vi "Main.vi"(11 "Args":string[](array[string])) -> (2 "Output":string, 3 "Exit Code":i32)   [LabVIEW 2021]
uses:
  <vilib>/Utility/config.llb/Read Key (String).vi
  <vilib>/Utility/file.llb/Write Delimited Spreadsheet (string).vi
  <vilib>/Utility/config.llb/Read Key (U32).vi
  Add_Library.lvlib
  <vilib>/Utility/config.llb/NI_LVConfig.lvlib
panel:
  in  "y":u64[](array[numeric])=[1, 2, 3]
  in  "x":u64[](array[numeric])=[1, 2, 3]
  out "x+y":u64[](array[numeric])
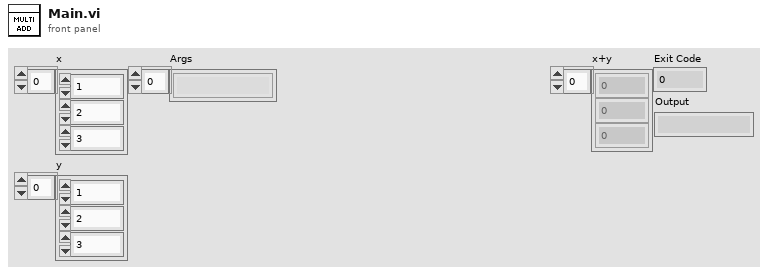
[diagram p1: front panel]
types:
  T1 = typedef "NI_LVConfig.lvlib/Config Data RefNum.ctl" = refnum<k1>
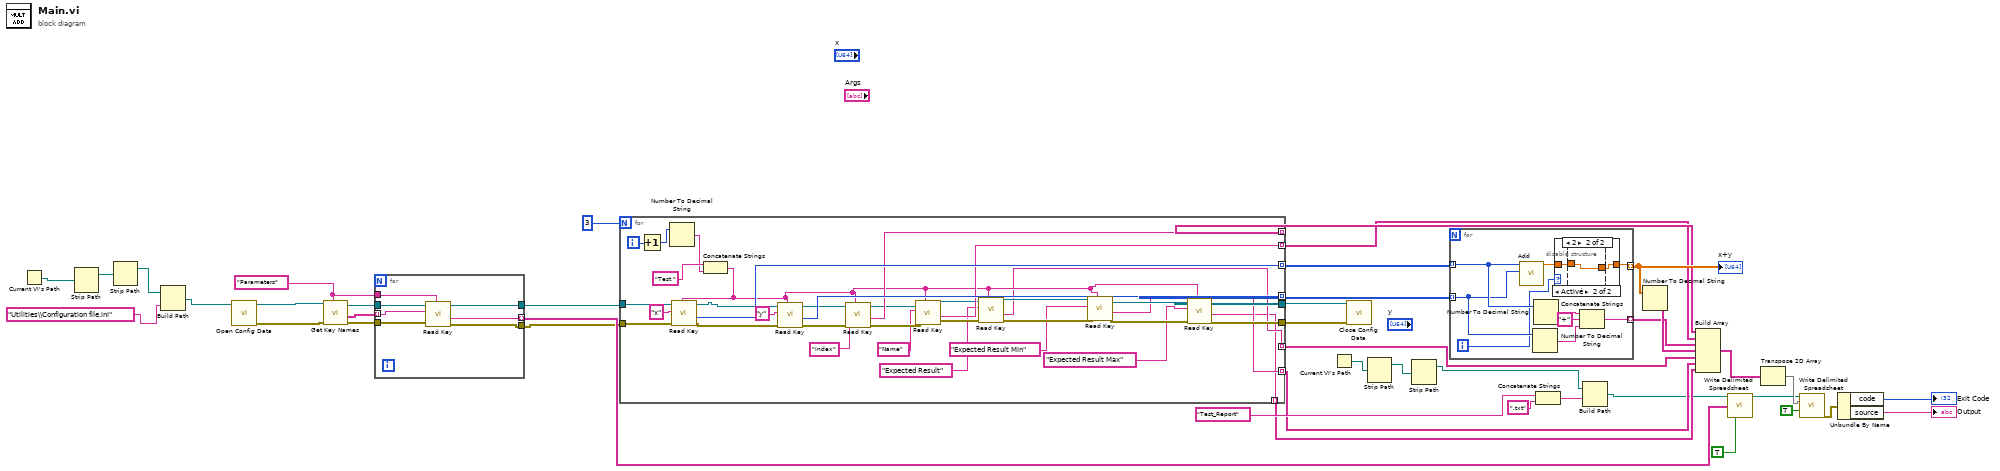
[diagram p0: block diagram]
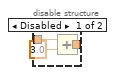
[diagram p3: hidden frame]
diagram:
  w8 = "Parameters" ("section")
  n1 = Current VI's Path() -> (path=w29:path)
  n2 = Strip Path(path=w29) -> (stripped path=w28:path)  [unwired: 1 out]
  n3 = Strip Path(path=w28) -> (stripped path=w27:path)  [unwired: 1 out]
  n4 = Build Path(base path=w27, name or relative path="Utilities\\Configuration file.ini" ("Report Path")) -> (appended path=w25:path)
  n5 = call <vilib>:"Open Config Data.vi"("configuration file path"=w25) -> ("error out"=w13:errorcluster, "refnum"=w14:T1)  [unwired: 8 in, 1 out]
  n6 = call <vilib>:"Get Key Names.vi"("section"=w8, "error in (no error)"=w13, "refnum"=w14) -> ("error out"=w10:errorcluster, "key names"=w9:string[], "refnum out"=w12:T1)  [unwired: 5 in, 1 out]
  n7 = for {
    tunnel: w12 -> [w49]
    tunnel: [w48] -> w11
    tunnel: w10 -> [w47]
    tunnel: w9 -> [w46] mode=indexing
    tunnel: w8 -> [w45]
    tunnel: [w44] -> w3 mode=indexing
    tunnel: [w43] -> w2
    n8 = call-poly <vilib>:"Read Key.vi"("section"=w45, "error in (no error)"=w47, "key"=w46, "refnum"=w49) -> ("error out"=w43:errorcluster, "value"=w44:string, "refnum out"=w48:T1)  [unwired: 4 in, 1 out]
  }
  n9 = for {
    N: 3 -> [_]
    tunnel: w2 -> [w84]
    tunnel: w11 -> [w83]
    tunnel: [w78] -> w24 mode=indexing
    tunnel: [w77] -> w23 mode=indexing
    tunnel: [w69] -> w21 mode=indexing
    tunnel: [w65] -> w20 mode=indexing
    tunnel: [w56] -> w19
    tunnel: [w55] -> w18
    tunnel: [w52] -> w17 mode=indexing
    tunnel: [w51] -> w16 mode=indexing
    tunnel: [w50] -> w15 mode=indexing
    i -> [w73]
    n10 = Increment(x=w73) -> (x+1=w74:i32)
    n11 = Number To Decimal String(number=w74) -> (decimal integer string=w75:string)  [unwired: 1 in]
    n12 = Concatenate Strings("Test " ("section"), w75) -> (w57:string)
    n13 = call-poly <vilib>:"Read Key.vi"("section"=w57, "error in (no error)"=w84, "key"="x", "refnum"=w83) -> ("error out"=w80:errorcluster, "value"=w78:u32, "refnum out"=w79:T1)  [unwired: 4 in, 1 out]
    n14 = call-poly <vilib>:"Read Key.vi"("section"=w57, "error in (no error)"=w80, "key"="y", "refnum"=w79) -> ("error out"=w72:errorcluster, "value"=w77:u32, "refnum out"=w71:T1)  [unwired: 4 in, 1 out]
    n15 = call-poly <vilib>:"Read Key.vi"("section"=w57, "error in (no error)"=w72, "key"="Index", "refnum"=w71) -> ("error out"=w68:errorcluster, "value"=w69:string, "refnum out"=w67:T1)  [unwired: 4 in, 1 out]
    n16 = call-poly <vilib>:"Read Key.vi"("section"=w57, "error in (no error)"=w68, "key"="Name", "refnum"=w67) -> ("error out"=w63:errorcluster, "value"=w65:string, "refnum out"=w64:T1)  [unwired: 4 in, 1 out]
    n17 = call-poly <vilib>:"Read Key.vi"("section"=w57, "error in (no error)"=w63, "key"="Expected Result", "refnum"=w64) -> ("error out"=w61:errorcluster, "value"=w52:string, "refnum out"=w62:T1)  [unwired: 4 in, 1 out]
    n18 = call-poly <vilib>:"Read Key.vi"("section"=w57, "error in (no error)"=w61, "key"="Expected Result Min", "refnum"=w62) -> ("error out"=w59:errorcluster, "value"=w51:string, "refnum out"=w58:T1)  [unwired: 4 in, 1 out]
    n19 = call-poly <vilib>:"Read Key.vi"("section"=w57, "error in (no error)"=w59, "key"="Expected Result Max", "refnum"=w58) -> ("error out"=w55:errorcluster, "value"=w50:string, "refnum out"=w56:T1)  [unwired: 4 in, 1 out]
  }
  n20 = Current VI's Path() -> (path=w38:path)
  n21 = call <vilib>:"Close Config Data.vi"("error in (no error)"=w18, "refnum"=w19) -> ()  [unwired: 8 in, 2 out]
  n22 = Strip Path(path=w38) -> (stripped path=w31:path)  [unwired: 1 out]
  n23 = Strip Path(path=w31) -> (stripped path=w30:path)  [unwired: 1 out]
  n24 = for {
    tunnel: w24 -> [w93] mode=indexing
    tunnel: w23 -> [w92] mode=indexing
    tunnel: [w86] -> w42 mode=indexing
    tunnel: [w88] -> w1 mode=indexing
    i -> [w85]
    n25 = call "Add.vi"("y"=w92, "x"=w93) -> ("x+y"=w87:dbl)  [unwired: 9 in]
    n26 = Number To Decimal String(number=w92) -> (decimal integer string=w89:string)  [unwired: 1 in]
    n27 = Number To Decimal String(number=w93) -> (decimal integer string=w91:string)  [unwired: 1 in]
    n28 = case shown="2" w85 {
      tunnel: w87 -> [w94 w96]
      tunnel: [w94 w95] -> w86
      frame 0, Default {
      }
      frame 2 {
        n29 = disable-structure shown="Activé" {
          disable-tunnel: w96 -> [w99 w100]
          disable-tunnel: [w97 w100] -> w95
          frame Disabled {
            n30 = Add(x=w99, y=3.0) -> (x+y=w97:dbl)
          }
          frame Enabled {
          }
        }
      }
    }
    n31 = Concatenate Strings(w91, "+" ("chaîne"), w89) -> (w88:string)
  }
  "x+y" <- w42
  n32 = Concatenate Strings("Test_Report" ("Report Path"), ".txt" ("chaîne")) -> (w37:string)
  n33 = Build Path(base path=w30, name or relative path=w37) -> (appended path=w5:path)
  n34 = Number To Decimal String(number=w42) -> (decimal integer string=w41:string[])  [unwired: 1 in]
  n35 = Build Array(w21, w20, w1, w41, w17, w16, w15) -> (w36:string[][])
  n36 = call-poly <vilib>:"Write Delimited Spreadsheet.vi"("file path (dialog if empty)"=w5, "1D data"=w3, "transpose? (no:F)"=TRUE) -> ("new file path (Not A Path if cancelled)"=w6:path)  [unwired: 11 in, 1 out]
  n37 = Transpose 2D Array(2D array=w36) -> (transposed array=w35:string[][])
  n38 = call-poly <vilib>:"Write Delimited Spreadsheet.vi"("file path (dialog if empty)"=w6, "2D data"=w35, "append to file? (new file:F)"=TRUE) -> ("error out"=w32:errorcluster)  [unwired: 11 in, 1 out]
  n39 = Unbundle By Name(w32) -> ("code"=→"Exit Code":i32, "source"=→"Output":string)
